vi "Release Delays.vi"(8 "error in (no error)":errorcluster, 11 "Release":bool) -> (0 "error out":errorcluster)   [LabVIEW 2009, in "POLARIS BME DG.lvlib"]
doc: "Deactivates the BME Delay Cards and frees the allocated memory.\nThomas Leisner Sept. 2001"
uses:
  POLARIS BME DG.lvlib
panel:
  # "NOTICE -- YOU MUST LEAVE THIS NOTICE IN PLACE.  PER THE TERMS OF THE LICENSE BELOW, YOU MAY SUBLICENSE THIS SOFTWARE \nIN ANY WAY THAT DOES NOT CONFLICT WITH THIS LICENSE.\n\n### BSD License (http://www.opensource.org/licenses/bsd-license.php) Begin ###\n \nCopyright (c) 2011, Applied Energetics, http://www.appliedenergetics.com,\n                               Richard Schwerdtfeger, <rschwerdtfeger@appliedenergetics.com>\n\nAll rights reserved.\n\nRedistribution and use in source and binary forms, with or without modification, are permitted provided that the \nfollowing conditions are met:\n\n    * Redistributions of source code must retain the above copyright notice, this list of conditions and the following disclaimer.\n    * Redistributions in binary form must reproduce the above copyright notice, this list of conditions and the following disclaimer \n       in the documentation and/or other materials provided with the distribution.\n    * Neither the name of Richard Schwerdtfeger, Applied Energetics, Inc., nor the names of its contributors may be used to \n       endorse or promote products derived from this software without specific prior written permission.\n\nTHIS SOFTWARE IS PROVIDED BY THE COPYRIGHT HOLDERS AND CONTRIBUTORS \"AS IS\" AND ANY EXPRESS OR IMPLIED WARRANTIES, \nINCLUDING, BUT NOT LIMITED TO, THE IMPLIED WARRANTIES OF MERCHANTABILITY AND FITNESS FOR A PARTICULAR PURPOSE ARE \nDISCLAIMED. IN NO EVENT SHALL THE COPYRIGHT OWNER OR CONTRIBUTORS BE LIABLE FOR ANY DIRECT, INDIRECT, INCIDENTAL,\n SPECIAL, EXEMPLARY, OR CONSEQUENTIAL DAMAGES (INCLUDING, BUT NOT LIMITED TO, PROCUREMENT OF SUBSTITUTE GOODS OR \nSERVICES; LOSS OF USE, DATA, OR PROFITS; OR BUSINESS INTERRUPTION) HOWEVER CAUSED AND ON ANY THEORY OF LIABILITY, \nWHETHER IN CONTRACT, STRICT LIABILITY, OR TORT (INCLUDING NEGLIGENCE OR OTHERWISE) ARISING IN ANY WAY OUT OF THE USE \nOF THIS SOFTWARE, EVEN IF ADVISED OF THE POSSIBILITY OF SUCH DAMAGE.\n\n### BSD License End ###"
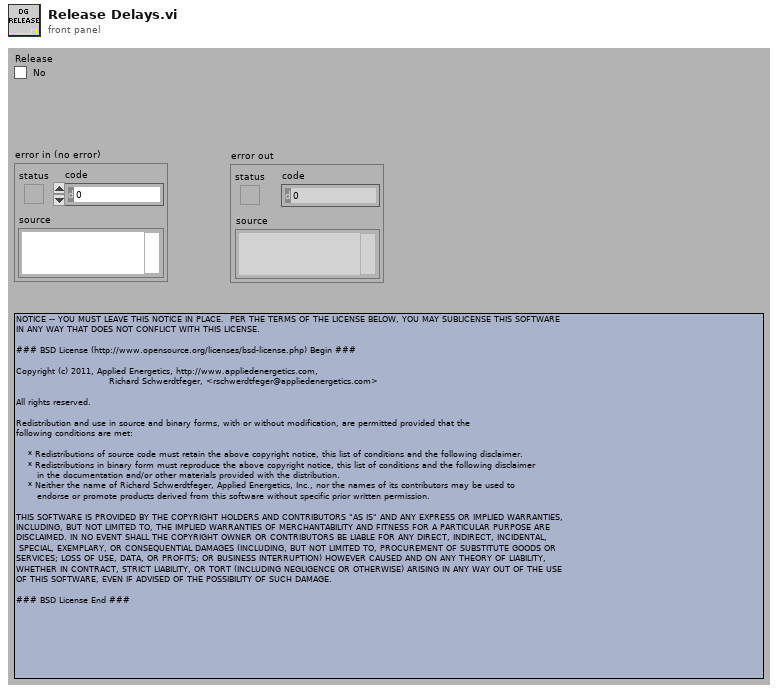
[diagram p1: front panel]
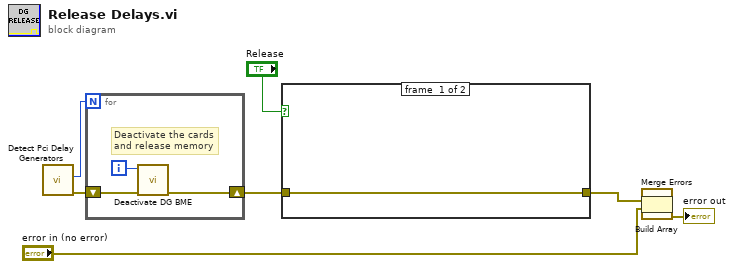
[diagram p0: block diagram]
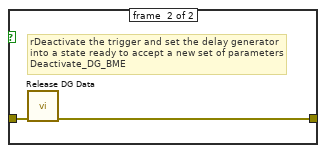
[diagram p2: hidden frame]
diagram:
  n1 = call "Detect Pci Delay Generators.vi"() -> ("error out"=w7:errorcluster, "Number of Generators"=w6:i32)  [unwired: 1 in, 9 out]
  n2 = for {
    N: w6 -> [_]
    shift-right: [w10] -> w8
    shift-left: w7 -> [w11]
    i -> [w9]
    # "Deactivate the cards \nand release memory"
    n3 = call "Deactivate DG BME.vi"("error in (no error)"=w11, "DG Number"=w9) -> ("error out"=w10:errorcluster)  [unwired: 9 out]
  }
  n4 = case shown="True" "Release" {
    tunnel: w8 -> [w12 w14]
    tunnel: [w12 w13] -> w3
    frame #0 {
    }
    frame #1 {
      # "rDeactivate the trigger and set the delay generator\ninto a state ready to accept a new set of parameters\nDeactivate_DG_BME"
      n5 = call "Release DG Data.vi"("error in (no error)"=w14) -> ("error out"=w13:errorcluster)  [unwired: 10 out]
    }
  }
  n6 = Build Array(w3, "error in (no error)") -> (w1:errorcluster[])
  n7 = call <vilib>:"Merge Errors.vi"("error array in"=w1) -> ("error out"=→"error out":errorcluster)  [unwired: 3 in, 3 out]
